vi "addSuccess.vi"(7 "execution time (sec)":dbl, 8 "error in (no error)":errorcluster, 10 "test":refnum<class>, 11 "TestTestResult in":refnum<class "_TextTestResult.lvclass">) -> (0 "error out":errorcluster, 3 "TestTestResult out":refnum<class "_TextTestResult.lvclass">)   [LabVIEW 2011, in "_TextTestResult.lvclass"]
uses:
  _TextTestResult.lvclass
  TestCase/TestCase.lvclass
  TestResult/TestResult.lvclass
  _TextTestResult.lvclass/_TextTestResult.ctl
panel:
  # "JKI VI Tester for LabVIEW\nhttp://jkisoft.com/vi-tester\nCopyright (C) 2007-2009, JKI <info@jkisoft.com>\nALL RIGHTS RESERVED"
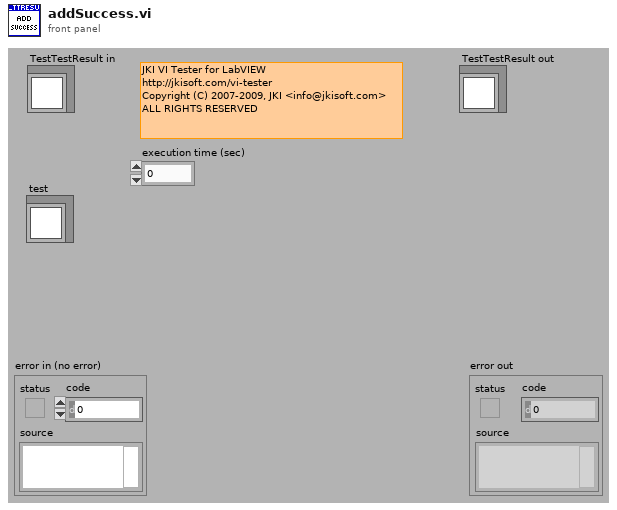
[diagram p1: front panel]
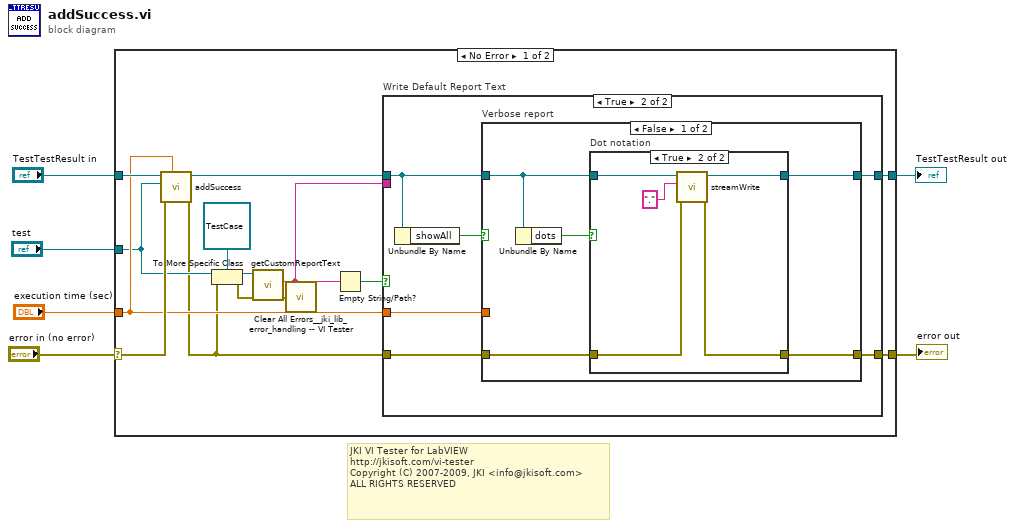
[diagram p0: block diagram]
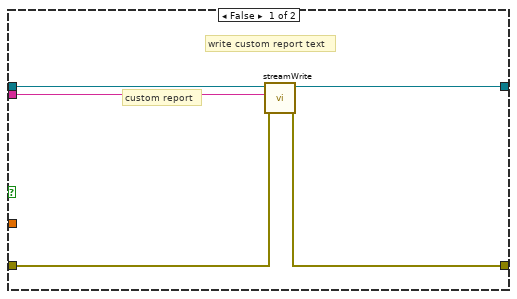
[diagram p2: hidden frame]
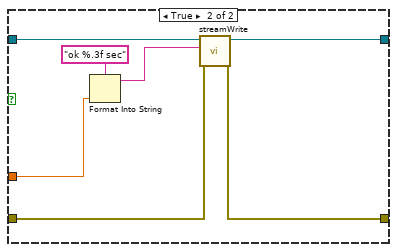
[diagram p4: hidden frame]
diagram:
  # "JKI VI Tester for LabVIEW\nhttp://jkisoft.com/vi-tester\nCopyright (C) 2007-2009, JKI <info@jkisoft.com>\nALL RIGHTS RESERVED"
  n1 = case shown="No Error" "error in (no error)" {
    selector: "error in (no error)" -> [w19 w52]
    tunnel: [w16 w52] -> w5
    tunnel: [w17 w51] -> w3
    tunnel: "TestTestResult in" -> [w20 w51]
    tunnel: "test" -> [w13 _]
    tunnel: "execution time (sec)" -> [w15 _]
    frame No Error {
      n2 = call-parent "addSuccess.vi"("execution time (sec)"=w15, "error in (no error)"=w19, "test"=w13, "TestResult in"=w20) -> ("error out"=w10:errorcluster, "TestResult in"=w18:refnum<class "_TextTestResult.lvclass">)  [unwired: 6 in]
      n3 = To More Specific Class(target class=refnum<class "TestCase.lvclass"> refnum ("TestCase in"), reference=w13, error in=w10) -> (specific class reference=w11:refnum<class "TestCase.lvclass">, error out=w14:errorcluster)
      n4 = call-dynamic "getCustomReportText.vi"("error in (no error)"=w14, "TestCase in"=w11) -> ("error out"=w9:errorcluster, "customReportText"=w7:string)  [unwired: 7 in, 1 out]
      n5 = call "Clear All Errors__jki_lib_error_handling -- VI Tester.vi"("error in"=w9) -> ()  [unwired: 4 in, 1 out]
      n6 = Empty String/Path?(string/path=w7) -> (empty?=w8:bool)
      n7 = case "Write Default Report Text" shown="True" w8 {
        tunnel: w18 -> [w25 w30]
        tunnel: [w24 w29] -> w17
        tunnel: [w22 w28] -> w16
        tunnel: w15 -> [_ w27]
        tunnel: w10 -> [w23 w26]
        tunnel: w7 -> [w21 _]
        frame False {
          # "custom report"
          # "write custom report text"
          n8 = call "streamWrite.vi"("error in (no error)"=w23, "String"=w21, "TestTestResult in"=w25) -> ("error out"=w22:errorcluster, "TestTestResult out"=w24:refnum<class "_TextTestResult.lvclass">)  [unwired: 7 in]
        }
        frame True {
          n9 = Unbundle By Name(w30) -> ("showAll"=w31:bool)
          n10 = case "Verbose report" shown="False" w31 {
            tunnel: w30 -> [w35 w50]
            tunnel: w26 -> [w33 w48]
            tunnel: [w32 w47] -> w28
            tunnel: [w36 w49] -> w29
            tunnel: w27 -> [_ w46]
            frame False {
              n11 = Unbundle By Name(w35) -> ("dots"=w34:bool)
              n12 = case "Dot notation" shown="True" w34 {
                tunnel: w35 -> [w37 w43]
                tunnel: w33 -> [w38 w40]
                tunnel: [w38 w39] -> w32
                tunnel: [w37 w42] -> w36
                frame False {
                }
                frame True {
                  n13 = call "streamWrite.vi"("error in (no error)"=w40, "String"="." ("element"), "TestTestResult in"=w43) -> ("error out"=w39:errorcluster, "TestTestResult out"=w42:refnum<class "_TextTestResult.lvclass">)  [unwired: 7 in]
                }
              }
            }
            frame True {
              n14 = Format Into String(format string="ok %.3f sec" ("element"), w46) -> (resulting string=w45:string)  [unwired: 2 in, 1 out]
              n15 = call "streamWrite.vi"("error in (no error)"=w48, "String"=w45, "TestTestResult in"=w50) -> ("error out"=w47:errorcluster, "TestTestResult out"=w49:refnum<class "_TextTestResult.lvclass">)  [unwired: 7 in]
            }
          }
        }
      }
    }
    frame Error {
    }
  }
  "error out" <- w5
  "TestTestResult out" <- w3
